vi "Grava_GlobalReg_u.vi"(2 "Global Register programmed":u32[](array[numeric])=[68228136, 235670073, 4294967264, 4294967295, 4294967295, 511] format="%x", 3 "Folder path":path) -> (1 "quants arxius fets":i32)   [LabVIEW 2015, in "VIPM2.lvlib"]
doc: "Grava els Global Registers programats en arxius personalitzats per ChipID\n\" \\ChipID_GlobalReg.txt \""
uses:
  VIPM2.lvlib
panel:
  # "Subrutina: grava els Global Registers programats en arxius personalitzats per ChipID"
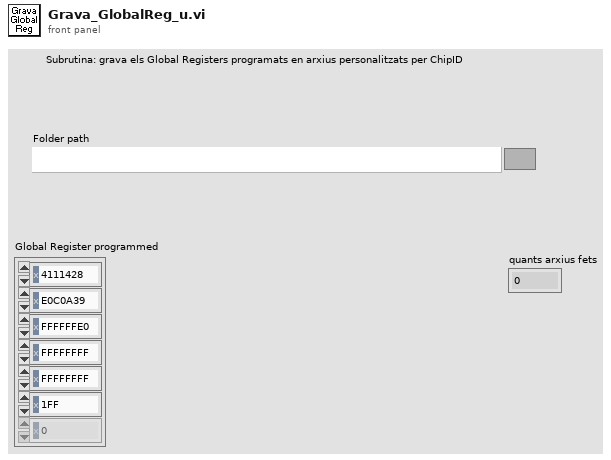
[diagram p1: front panel]
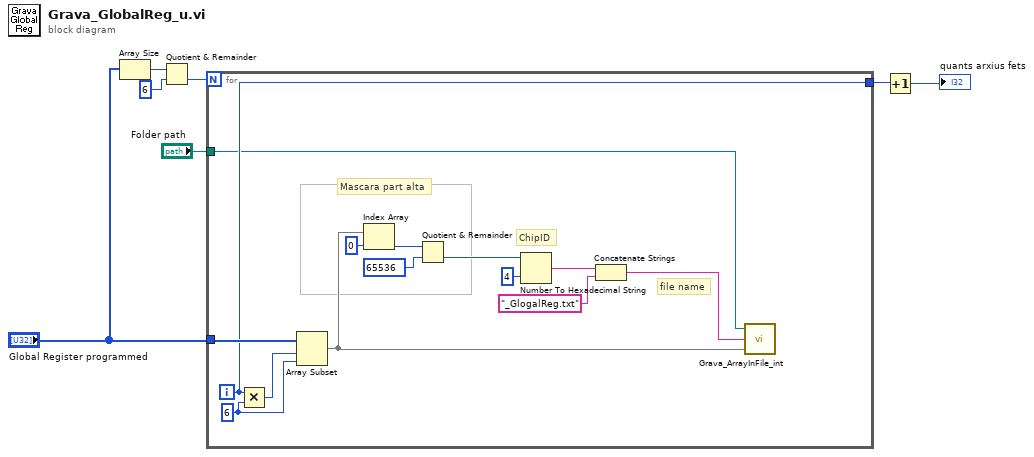
[diagram p0: block diagram]
diagram:
  n1 = Array Size(array="Global Register programmed") -> (size(s)=w6:i32)
  n2 = Quotient & Remainder(x=w6, y=6) -> (floor(x/y)=w7:i32)  [unwired: 1 out]
  n3 = for {
    N: w7 -> [_]
    tunnel: "Global Register programmed" -> [w21]
    tunnel: [w11] -> w3
    tunnel: "Folder path" -> [w9]
    i -> [w11]
    w19 = 6 ("y")
    # "file name"
    # "ChipID"
    # "Mascara part alta"
    n4 = Multiply(x=w11, y=w19) -> (x*y=w20:i32)
    n5 = Array Subset "Array Subset"(array=w21, index=w20, length=w19) -> (w10:u32[])
    n6 = Index Array "Index Array"(array=w10, index=0) -> (element=w17:u32)
    n7 = Quotient & Remainder(x=w17, y=u32 65536) -> (floor(x/y)=w15:u32)  [unwired: 1 out]
    n8 = Number To Hexadecimal String(1:i16 4 ("width (-)"), 2:w15) -> (0:w13:string)
    n9 = Concatenate Strings "Concatenate Strings"(w13, "_GlogalReg.txt" ("string")) -> (w8:string)
    n10 = call "Grava_ArrayInFile_int.vi"("Array to save"=w10, "file name"=w8, "folder path"=w9) -> ()  [unwired: 2 in]
  }
  n11 = Increment(x=w3) -> (x+1=→"quants arxius fets":i32)
